vi "Waveform Attribute, Get All Atttributes.vi"(6 "error in":errorcluster, 9 "waveform":waveform(dbl)={"t0"=timestamp(3473168117.0530005 s since 1904-01-01), "dt"=4e-06, "Y"=[], "attributes"=variant("Average Size"=variant(dbl 15.0), "Frequency (Hz)"=variant(dbl 1.998745962823557), "Number of Samples"=variant(dbl 750000.0), "Process Timestamp"=variant(timestamp timestamp(3474401815.53125 s since 1904-01-01)), "Recvy Amp (V)"=variant(dbl 5.120123508943166), "Recvy Amp (mA)"=variant(dbl 10.240247017886333), "Recvy Frequency (Hz)"=variant(dbl 1.9987453162428834), "Recvy Pulse Width (us)"=variant(dbl 422.33480072021484), "Recvy Trigger (s)"=variant(dbl 0.35626399999999997), "Resistance (ohms)"=variant(dbl 500.0), "Sample Frequency (MHz)"=variant(dbl 0.25), "Stim Amp (V)"=variant(dbl -4.84918832438602), "Stim Amp (mA)"=variant(dbl -9.698376648772038), "Stim Frequency (Hz)"=variant(dbl 1.9987466094042308), "Stim Pulse Width (us)"=variant(dbl 417.8791389465332), "Stim Trigger (s)"=variant(dbl 0.355772), "dt (us)"=variant(dbl 4.0))}) -> (0 "error out":errorcluster, 2 "all attributes":T1[](array[typedef]) {"Value" format="%#.3f"}, 3 "waveform dup":waveform(dbl)={"t0"=timestamp(0 s since 1904-01-01), "dt"=nan, "Y"=[]})   [LabVIEW 2010]
doc: "This function attempts to get all of the waveform attribute labels and values.\n\nAny waveform attributes that can't be converted are not appended and will not cause an error."
uses:
  Waveform Attribute Cluster.ctl
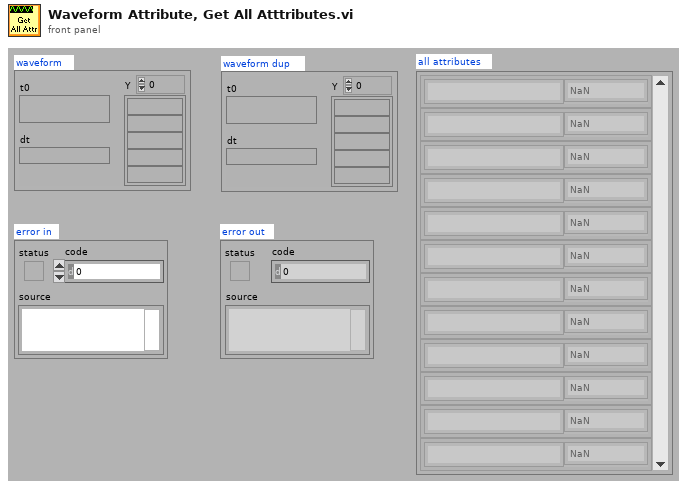
[diagram p1: front panel]
types:
  T1 = typedef "Waveform Attribute Cluster.ctl" = cluster{"Label":string, "Value":dbl}
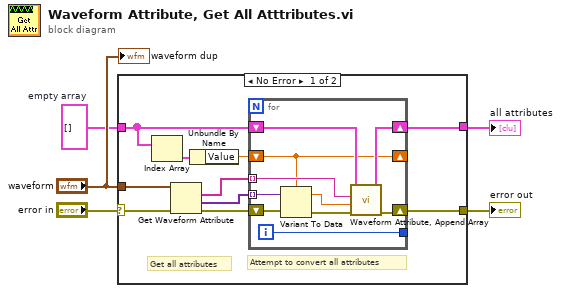
[diagram p0: block diagram]
diagram:
  w3 = cluster{"Label":string, "Value":dbl}[] []  # empty array
  n1 = case shown="No Error" "error in" {
    selector: "error in" -> [w9 w27]
    tunnel: "waveform" -> [w13 _]
    tunnel: [w12 w27] -> w1
    tunnel: w3 -> [w8 w26]
    tunnel: [w11 w26] -> w2
    frame No Error {
      # "Attempt to convert all attributes"
      # "Get all attributes"
      n2 = Index Array(array=w8) -> (element=w7:cluster{"Label":string, "Value":dbl})  [unwired: 1 in]
      n3 = Get Waveform Attribute(4:w9, 7:w13) -> (0:w14:errorcluster, 1:w10:variant[], 2:w15:string[])  [unwired: 2 in, 1 out]
      n4 = Unbundle By Name(w7) -> ("Value"=w6:dbl)
      n5 = for {
        tunnel: w15 -> [w21] mode=indexing
        tunnel: w10 -> [w25] mode=indexing
        shift-right: [w19] -> w12
        shift-left: w14 -> [w24]
        shift-right: [w20] -> w11
        shift-left: w8 -> [w18]
        tunnel: [w17] -> _
        shift-right: [w16] -> _
        shift-left: w6 -> [w16]
        i -> [w17]
        n6 = Variant To Data(error in=w24, Variant=w25, type=w16) -> (error out=w23:errorcluster, data=w22:dbl)
        n7 = call "Waveform Attribute, Append Array.vi"("error in"=w23, "value"=w22, "label"=w21, "attributes"=w18) -> ("error out"=w19:errorcluster, "attributes out"=w20:T1[])  [unwired: 4 in]
      }
    }
    frame Error {
    }
  }
  "error out" <- w1
  "all attributes" <- w2
  "waveform dup" <- "waveform"
